vi "toJSON.vi"(8 "error in (no error)":errorcluster, 11 "tBSONTimestamp in":refnum<class "tBSONTimestamp.lvclass">) -> (0 "error out":errorcluster, 2 "JSON":string, 3 "tBSONTimestamp out":refnum<class "tBSONTimestamp.lvclass">)   [LabVIEW 2013, in "BSON.lvlib" / "tBSONTimestamp.lvclass"]
uses:
  tBSONTimestamp.lvclass
  tBSONElement/tBSONElement.lvclass
  getValue.vi
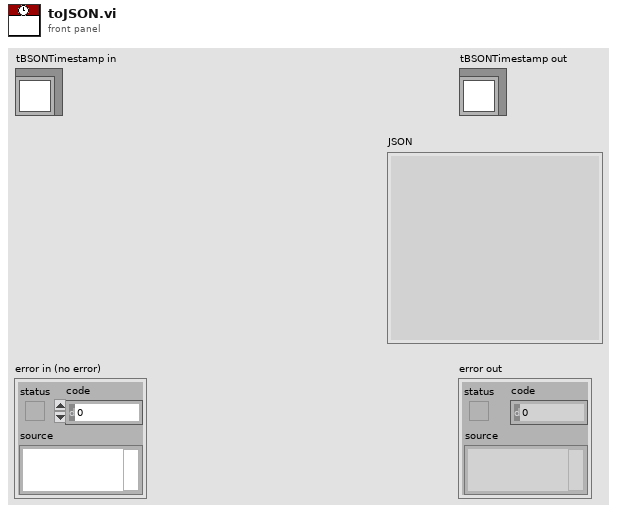
[diagram p1: front panel]
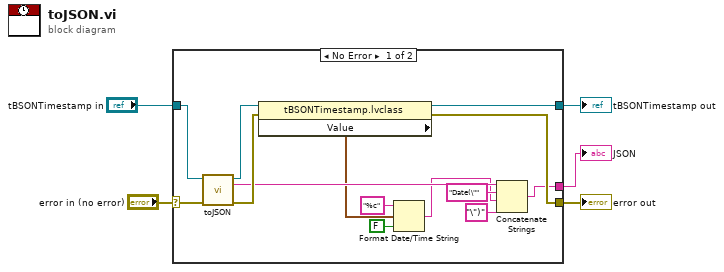
[diagram p0: block diagram]
diagram:
  n1 = case shown="No Error" "error in (no error)" {
    selector: "error in (no error)" -> [w18 w20]
    tunnel: [w14 w20] -> w5
    tunnel: [w6 _] -> w4
    tunnel: "tBSONTimestamp in" -> [w19 w21]
    tunnel: [w15 w21] -> w2
    frame No Error {
      n2 = call-parent "toJSON.vi"("error in (no error)"=w18, "tBSONElement in"=w19) -> ("error out"=w16:errorcluster, "JSON"=w13:string, "tBSONElement out"=w17:refnum<class "tBSONTimestamp.lvclass">)  [unwired: 7 in]
      n3 = property class="tBSONTimestamp.lvclass"(reference=w17, error in=w16) -> (reference out=w15:refnum<class "tBSONTimestamp.lvclass">, error out=w14:errorcluster, "Value"=w10:timestamp)
      n4 = Format Date/Time String(time format string (%c)="%c", seconds (now)=w10, UTC format=FALSE) -> (date/time string=w7:string)
      n5 = Concatenate Strings(w13, "Date(\"" ("string"), w7, "\")" ("string")) -> (w6:string)
    }
    frame Error {
    }
  }
  "error out" <- w5
  "tBSONTimestamp out" <- w2
  "JSON" <- w4
